vi "S1500_BCDtoDEZIMAL.vi"(10 "BCD BYTE":u8) -> (2 "Dezimal":i32)   [LabVIEW 2018]
panel:
  out "Zehner":u32
  out "Einer":u32
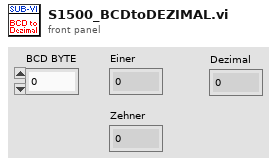
[diagram p1: front panel]
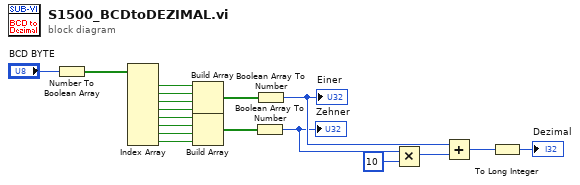
[diagram p0: block diagram]
diagram:
  n1 = Number To Boolean Array(number="BCD BYTE") -> (Boolean array=w4:bool[])
  n2 = Index Array(array=w4) -> (element #1=w5:bool, element #2=w6:bool, element #3=w7:bool, element #4=w8:bool, element #5=w11:bool, element #6=w12:bool, element #7=w13:bool, element #8=w14:bool)  [unwired: 8 in]
  n3 = Build Array(w5, w6, w7, w8) -> (w9:bool[])
  n4 = Build Array(w11, w12, w13, w14) -> (w10:bool[])
  n5 = Boolean Array To Number(Boolean array=w10) -> (number=w15:u32)
  "Zehner" <- w15
  n6 = Boolean Array To Number(Boolean array=w9) -> (number=w18:u32)
  "Einer" <- w18
  n7 = Multiply(x=w15, y=u32 10) -> (x*y=w17:u32)
  n8 = Add(x=w18, y=w17) -> (x+y=w2:u32)
  n9 = To Long Integer(number=w2) -> (32bit integer=→"Dezimal":i32)
